vi "General_TransferPoint_CT.vi"(10 "Coordinate":dbl[](array[numeric])=[0.0, 0.0, 0.0]) -> (2 "Command":string)   [LabVIEW 2017]
uses:
  sobot structures/SoBot_CommandTypes.ctl
  sobot structures/General_Command.ctl
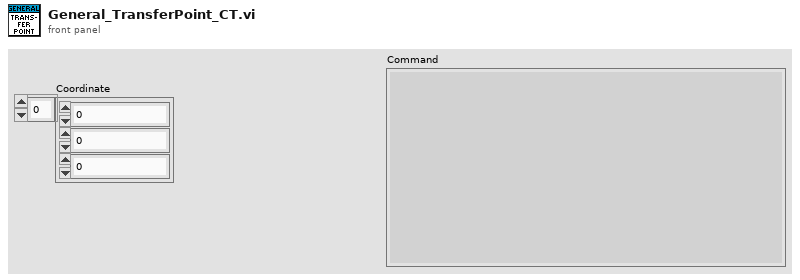
[diagram p1: front panel]
types:
  T1 = typedef "General_Command.ctl" = enum16{"General_Stop", "General_StartSobotAutomatic", "General_StopSobotAutomatic", "General_TransferPoint", "General_Initialize", "General_SimpleMessage", "General_Ping"}
  T2 = typedef "SoBot_CommandTypes.ctl" = enum16{"General_Command", "XY_Command", "Z_Command", "Plattform_Command"}
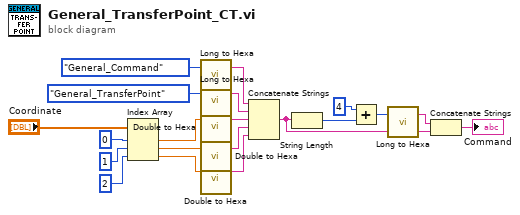
[diagram p0: block diagram]
diagram:
  n1 = Index Array(array="Coordinate", index #1=0 ("index"), index #2=1 ("index"), index #3=2 ("index")) -> (element #1=w10:dbl, element #2=w5:dbl, element #3=w4:dbl)
  n2 = call "Long to Hexa.vi"("Long"=SoBot_CommandTypes."General_Command" ("SoBot_CommandTypes")) -> ("Hexa"=w20:string)  [unwired: 2 in]
  n3 = call "Long to Hexa.vi"("Long"=General_Command."General_TransferPoint" ("General_Command")) -> ("Hexa"=w19:string)  [unwired: 2 in]
  n4 = call "Double to Hexa.vi"("Double"=w10) -> ("Hexa"=w3:string)  [unwired: 2 in]
  n5 = call "Double to Hexa.vi"("Double"=w5) -> ("Hexa"=w2:string)  [unwired: 2 in]
  n6 = call "Double to Hexa.vi"("Double"=w4) -> ("Hexa"=w1:string)  [unwired: 2 in]
  n7 = Concatenate Strings(w20, w19, w3, w2, w1) -> (w14:string)
  n8 = String Length(string=w14) -> (length=w18:i32)
  n9 = Add(x=4, y=w18) -> (x+y=w16:i32)
  n10 = call "Long to Hexa.vi"("Long"=w16) -> ("Hexa"=w15:string)  [unwired: 2 in]
  n11 = Concatenate Strings(w15, w14) -> (→"Command":string)
